vi "example_discrete.vi"() -> ()   [LabVIEW 2021, in "libad4.lvlib"]
uses:
  <userlib>/libad4/libad4.lvlib
panel:
  in  "Discrete - Analog Channel 1 and 2":dbl[](array[numeric])
  out "Discrete - Analog Channel 1 and 2":u64[](array[numeric])
  out "Discrete - Analog Channel 1 64bit":dbl
  out "Discrete - Analog Channel 1":sgl
  in  "DAQ ID":string
  in  "Discrete - Analog Channel 1 64bit":dbl
  in  "Discrete - Analog Channel 1":sgl
  in  "Digital Output - Channel 1":u32
  in  "Analog Output - Channel 1":sgl
  in  "Set button":bool
  out "Digital - Channel 1":u32
  out "Analog - Channel 1":sgl
  in  "Read button":bool
  # "DAQ Inputs"
  # "DAQ Outputs"
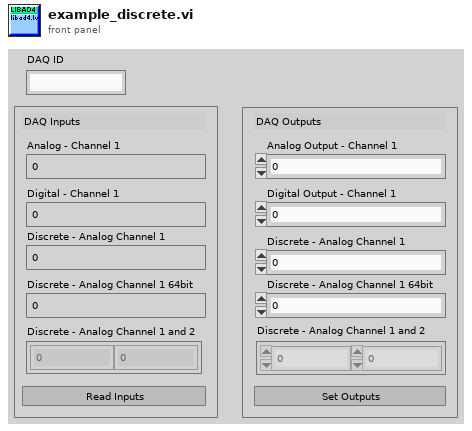
[diagram p1: front panel]
types:
  T1 = enum16{"AD_CHA_TYPE_ANALOG_IN", "AD_CHA_TYPE_ANALOG_OUT", "AD_CHA_TYPE_DIGITAL_IO"}
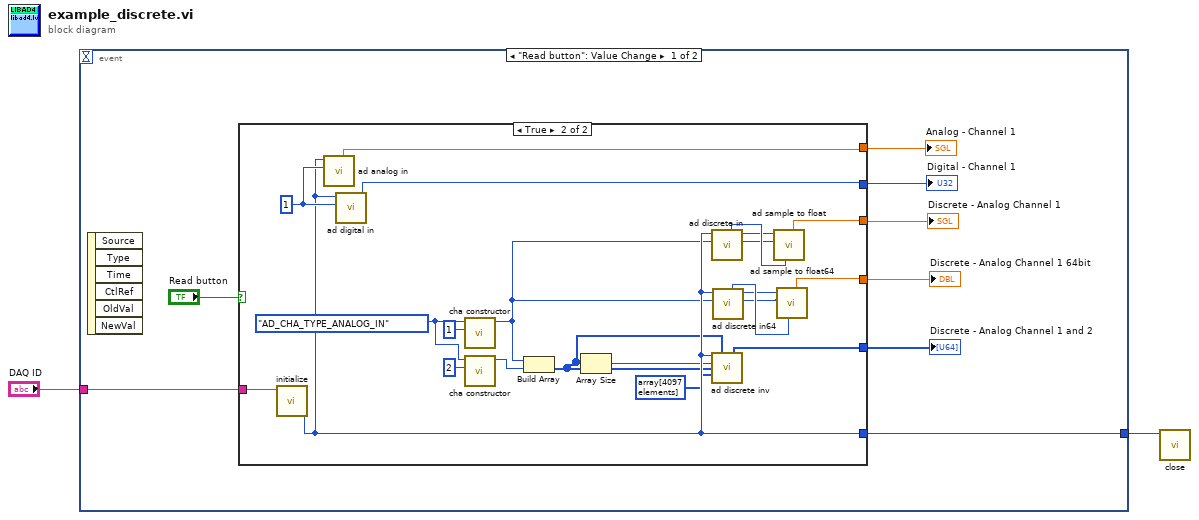
[diagram p0: block diagram]
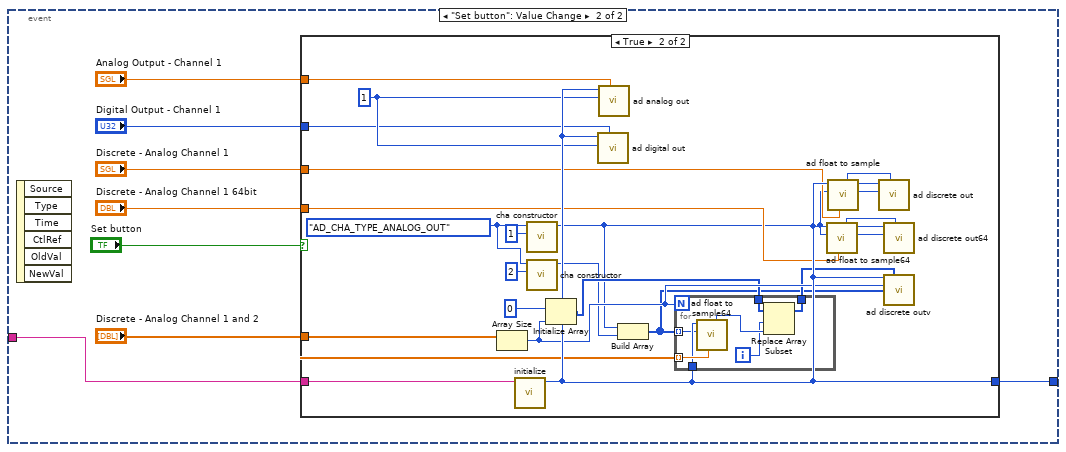
[diagram p3: hidden frame]
diagram:
  n1 = event shown="[0] \"Read button\": Value Change" {
    selector: _ -> [_ _]
    dyn-events: _ -> [_ _]
    timeout: _ -> [_ _]
    tunnel: [w9 w36] -> w2
    tunnel: "DAQ ID" -> [w6 w35]
    event "Read button": Value Change {
      n2 = event-data() -> ()  [unwired: 1 in, 6 out]
      n3 = case shown="True" "Read button" {
        tunnel: [_ w28] -> w7
        tunnel: [_ w25] -> w5
        tunnel: [_ w27] -> w8
        tunnel: [_ w20] -> w9
        tunnel: w6 -> [_ w26]
        tunnel: [_ w22] -> w4
        tunnel: [_ w12] -> w3
        frame False {
        }
        frame True {
          w17 = T1."AD_CHA_TYPE_ANALOG_IN" ("Channel Type")
          w21 = 1
          n4 = call <userlib>:"initialize.vi"("name"=w26) -> ("function return"=w20:i32)  [unwired: 9 in, 1 out]
          n5 = call <userlib>:"ad analog in.vi"("cha"=w21, "adh"=w20) -> ("data out"=w28:sgl)  [unwired: 7 in, 2 out]
          n6 = call <userlib>:"ad digital in.vi"("cha"=w21, "adh"=w20) -> ("data out"=w27:u32)  [unwired: 7 in, 2 out]
          n7 = call <userlib>:"cha constructor.vi"("Channel No."=1, "Channel Type"=w17) -> ("Channel Number"=w15:i32)  [unwired: 9 in]
          n8 = call <userlib>:"cha constructor.vi"("Channel No."=2, "Channel Type"=w17) -> ("Channel Number"=w16:i32)  [unwired: 9 in]
          n9 = Build Array(w15, w16) -> (w11:i32[])
          n10 = Array Size(array=w11) -> (size(s)=w14:i32)
          n11 = call <userlib>:"ad discrete in.vi"("cha"=w15, "adh"=w20) -> ("data out"=w24:u32)  [unwired: 7 in, 2 out]
          n12 = call <userlib>:"ad discrete inv.vi"("adh"=w20, "datav"=w11, "chac"=w14, "chav"=w11, "rangev"=u64[] array[4097 elements]) -> ("datav out"=w12:u64[])  [unwired: 8 in, 2 out]
          n13 = call <userlib>:"ad discrete in64.vi"("cha"=w15, "adh"=w20) -> ("data out"=w23:u64)  [unwired: 7 in, 2 out]
          n14 = call <userlib>:"ad sample to float.vi"("data"=w24, "cha"=w15, "adh"=w20) -> ("dbl out"=w25:sgl)  [unwired: 6 in, 2 out]
          n15 = call <userlib>:"ad sample to float64.vi"("data"=w23, "cha"=w15, "adh"=w20) -> ("dbl out"=w22:dbl)  [unwired: 6 in, 2 out]
        }
      }
      "Analog - Channel 1" <- w7
      "Digital - Channel 1" <- w8
      "Discrete - Analog Channel 1" <- w5
      "Discrete - Analog Channel 1 64bit" <- w4
      "Discrete - Analog Channel 1 and 2" <- w3
    }
    event "Set button": Value Change {
      n16 = event-data() -> ()  [unwired: 1 in, 6 out]
      n17 = case shown="True" "Set button" {
        tunnel: [_ w53] -> w36
        tunnel: w35 -> [_ w56]
        tunnel: "Discrete - Analog Channel 1 and 2" -> [_ w46]
        tunnel: "Discrete - Analog Channel 1 64bit" -> [_ w45]
        tunnel: "Discrete - Analog Channel 1" -> [_ w44]
        tunnel: "Digital Output - Channel 1" -> [_ w43]
        tunnel: "Analog Output - Channel 1" -> [_ w42]
        frame False {
        }
        frame True {
          w37 = T1."AD_CHA_TYPE_ANALOG_OUT" ("Channel Type")
          w51 = 1
          n18 = Array Size(array=w46) -> (size(s)=w52:i32)
          n19 = call <userlib>:"initialize.vi"("name"=w56) -> ("function return"=w53:i32)  [unwired: 9 in, 1 out]
          n20 = call <userlib>:"cha constructor.vi"("Channel No."=1, "Channel Type"=w37) -> ("Channel Number"=w41:i32)  [unwired: 9 in]
          n21 = call <userlib>:"cha constructor.vi"("Channel No."=2, "Channel Type"=w37) -> ("Channel Number"=w40:i32)  [unwired: 9 in]
          n22 = Initialize Array(u64 0, w52) -> (w50:u64[])
          n23 = call <userlib>:"ad digital out.vi"("data"=w43, "cha"=w51, "adh"=w53) -> ()  [unwired: 7 in, 2 out]
          n24 = call <userlib>:"ad analog out.vi"("data"=w42, "cha"=w51, "adh"=w53) -> ()  [unwired: 7 in, 2 out]
          n25 = Build Array(w41, w40) -> (w47:i32[])
          n26 = for {
            N: w52 -> [_]
            tunnel: w46 -> [w63] mode=indexing
            tunnel: w53 -> [w62]
            tunnel: w47 -> [w61] mode=indexing
            tunnel: w50 -> [w59]
            tunnel: [w57] -> w48
            i -> [w58]
            n27 = call <userlib>:"ad float to sample64.vi"("dbl"=w63, "cha"=w61, "adh"=w62) -> ("sample out"=w60:u64)  [unwired: 6 in, 2 out]
            n28 = Replace Array Subset(array=w59, new element=w60, index=w58) -> (w57:u64[])
          }
          n29 = call <userlib>:"ad float to sample64.vi"("dbl"=w45, "cha"=w41, "adh"=w53) -> ("sample out"=w55:u64)  [unwired: 6 in, 2 out]
          n30 = call <userlib>:"ad float to sample.vi"("dbl"=w44, "cha"=w41, "adh"=w53) -> ("sample out"=w54:u32)  [unwired: 6 in, 2 out]
          n31 = call <userlib>:"ad discrete out.vi"("data"=w54, "cha"=w41, "adh"=w53) -> ()  [unwired: 7 in, 2 out]
          n32 = call <userlib>:"ad discrete out64.vi"("data"=w55, "cha"=w41, "adh"=w53) -> ()  [unwired: 7 in, 2 out]
          n33 = call <userlib>:"ad discrete outv.vi"("adh"=w53, "datav"=w48, "chac"=w52, "chav"=w47) -> ()  [unwired: 10 in, 2 out]
        }
      }
    }
  }
  n34 = call <userlib>:"close.vi"("adh"=w2) -> ()  [unwired: 9 in, 2 out]
